vi "New Report Page.vi"(0 "report in":refnum<class "NI_Standard Report.lvclass">, 9 "MS Office parameters":T1, 11 "error in (no error)":errorcluster) -> (4 "report out":refnum<class "NI_Standard Report.lvclass">, 15 "error out":errorcluster)   [LabVIEW 2015, in "NI_Standard Report.lvclass"]
doc: "Creates a page break within the report. You cannot use this VI with HTML reports."
uses:
  <vilib>/Utility/NIReport.llb/Standard Report/NI_Standard Report.lvclass
  <vilib>/Utility/NIReport.llb/Standard Report/NI_Standard Report.lvclass/NI_Standard Report.ctl
  <vilib>/Utility/NIReport.llb/NI_ReportGenerationCore.lvlib
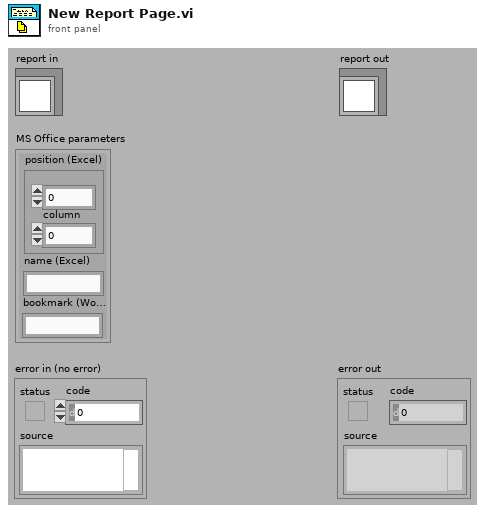
[diagram p1: front panel]
types:
  T1 = cluster{"position (Excel)":cluster{"row":i32, "column":i32}, "name (Excel) ":string, "bookmark (Word)":string}
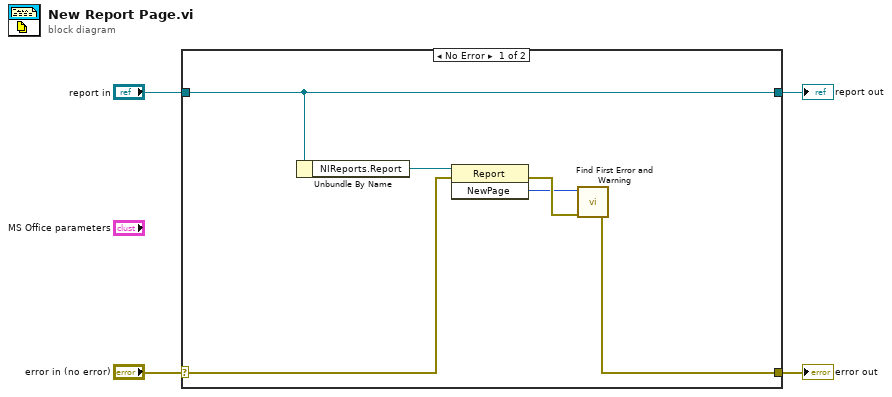
[diagram p0: block diagram]
diagram:
  n1 = case shown="No Error" "error in (no error)" {
    selector: "error in (no error)" -> [w6 w12]
    tunnel: [w5 w12] -> w3
    tunnel: [w7 w11] -> w1
    tunnel: "report in" -> [w7 w11]
    frame No Error {
      n2 = Unbundle By Name(w7) -> ("NIReports.Report"=w10:refnum<k7>)
      n3 = invoke class="Report" method="NewPage"(reference=w10, error in=w6) -> (error out=w9:errorcluster, "NewPage"=w8:i32)  [unwired: 1 in, 1 out]
      n4 = call <vilib>:"Find First Error and Warning.vi"("error in (no error)"=w9, "error code"=w8) -> ("error out"=w5:errorcluster)  [unwired: 1 in, 4 out]
    }
    frame Error {
    }
  }
  "error out" <- w3
  "report out" <- w1
